vi "Average_Block_Timetraces.vi"() -> (5 "Plug in titles":string[](array[string]), 7 "Plug in values":string[](array[string]))   [LabVIEW 2012]
uses:
  Globals/Meas_global.vi
panel:
  out "Current Block No":i32=51
  out "XY Graph":cluster{"Time (s)":dbl[], "Eng Values":dbl[]}[](graph)
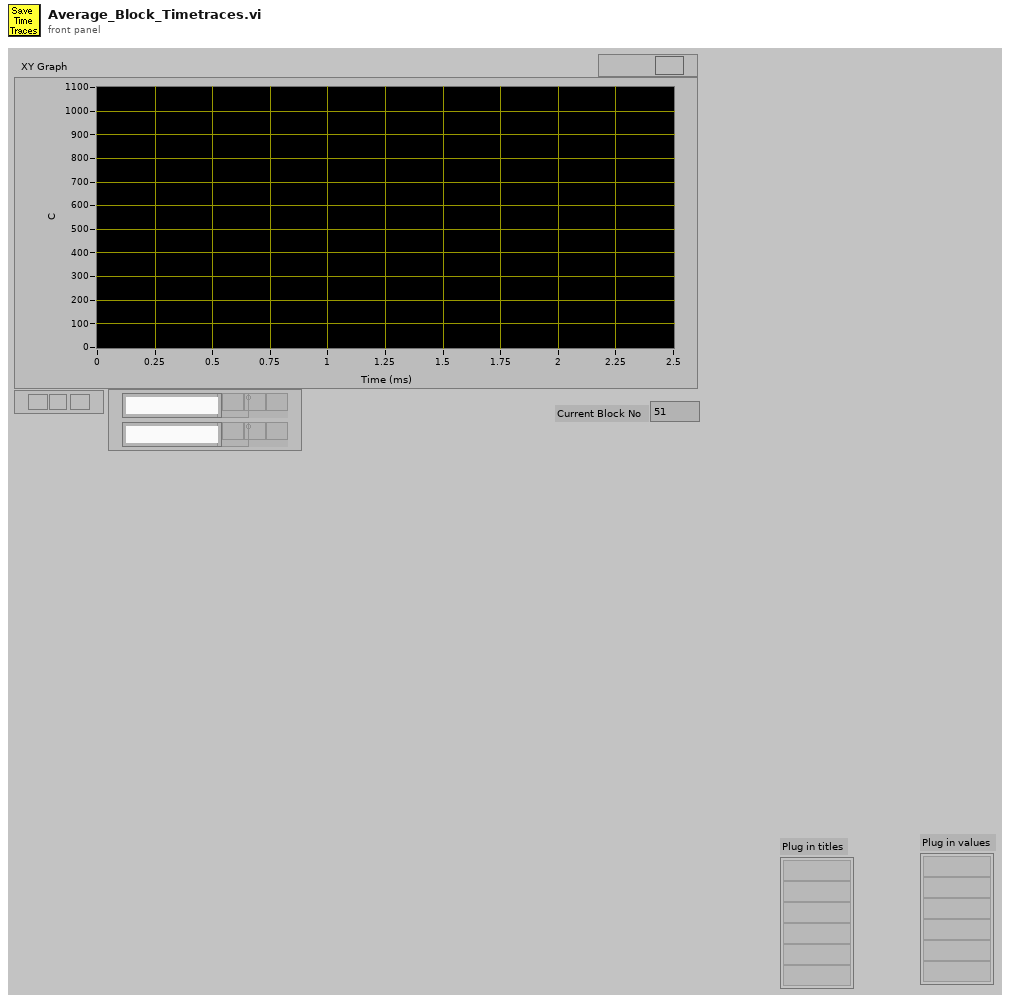
[diagram p1: front panel]
types:
  T1 = typedef "Time_Trace_Cluster.ctl" = cluster{"Weighting":dbl[], "Time (s)":dbl[], "Voltage":dbl[], "Eng Values":dbl[]}
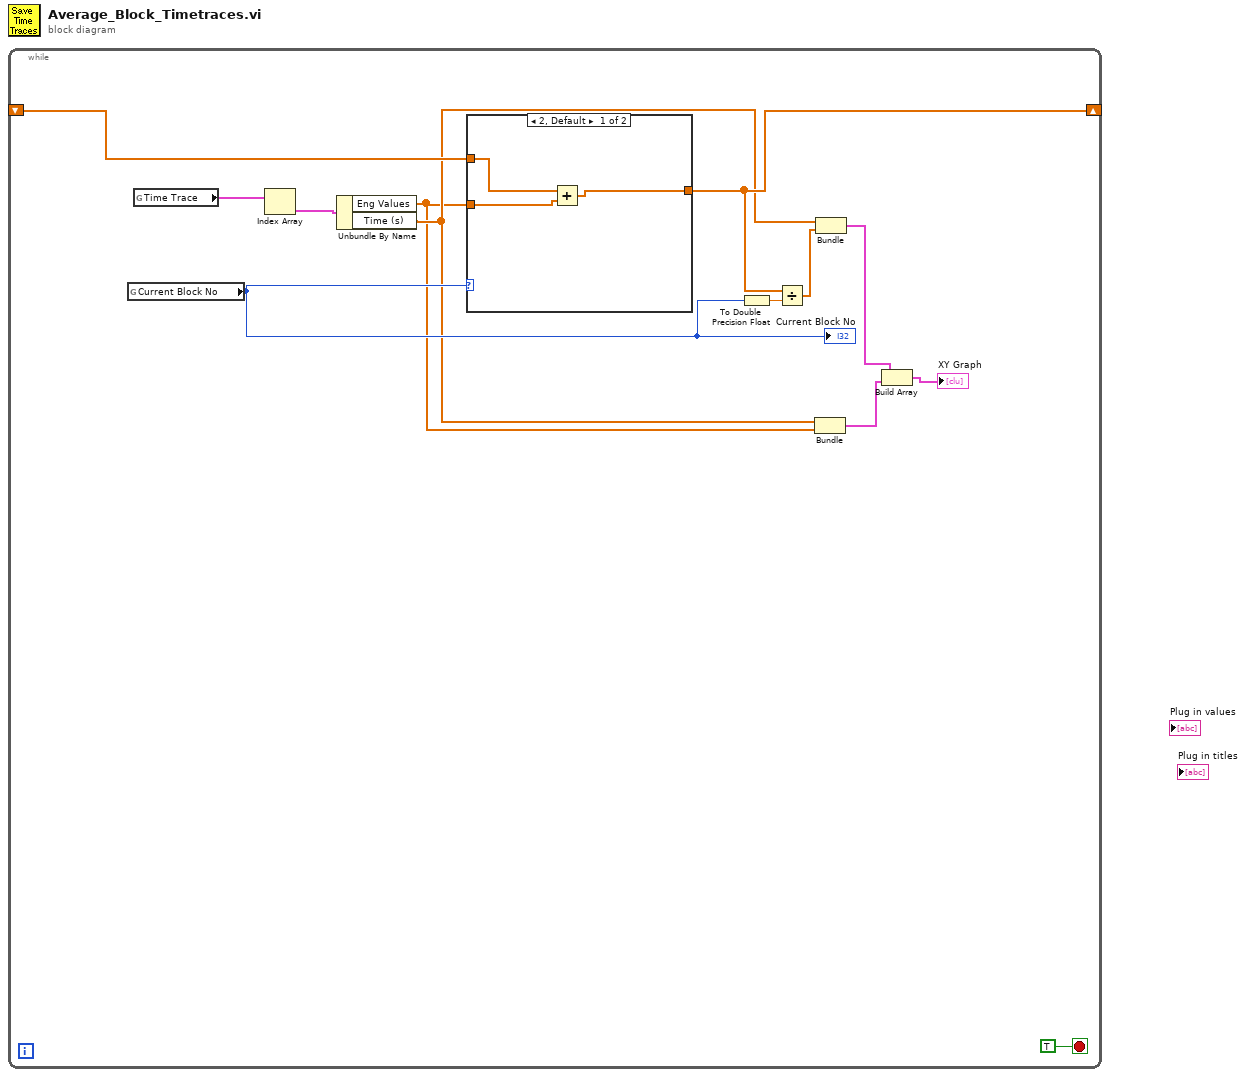
[diagram p0: block diagram]
diagram:
  n1 = while {
    shift-right: [w8] -> _
    shift-left: _ -> [w12]
    stop <- TRUE stop-if-true
    n2 = global read "Meas_global.vi" "Current Block No"() -> (w9:i32)
    "Current Block No" <- w9
    n3 = global read "Meas_global.vi" "Time Trace"() -> (w13:T1[])
    n4 = Index Array(array=w13) -> (element=w6:T1)  [unwired: 1 in]
    n5 = Unbundle By Name(w6) -> ("Eng Values"=w4:dbl[], "Time (s)"=w5:dbl[])
    n6 = case shown="2, Default" w9 {
      tunnel: [w14 w17] -> w8
      tunnel: w4 -> [w16 w17]
      tunnel: w12 -> [w15 _]
      frame 2, Default {
        n7 = Add(x=w15, y=w16) -> (x+y=w14:dbl[])
      }
      frame 1 {
      }
    }
    n8 = To Double Precision Float(number=w9) -> (double precision float=w10:dbl)
    n9 = Divide(x=w8, y=w10) -> (x/y=w7:dbl[])
    n10 = Bundle("Time (s)"=w5, "Eng Values"=w4) -> (w3:cluster{"Time (s)":dbl[], "Eng Values":dbl[]})  [unwired: 1 in]
    n11 = Bundle("Time (s)"=w5, w7) -> (w2:cluster{"Time (s)":dbl[], dbl[]})  [unwired: 1 in]
    n12 = Build Array(w2, w3) -> (→"XY Graph":cluster{"Time (s)":dbl[], "Eng Values":dbl[]}[])
  }
